vi "write checkpoint report.vi"(8 "error in (no error)":errorcluster, 11 "Autofocus in":refnum<class "Autofocus.lvclass">) -> (0 "error out":errorcluster, 3 "Autofocus out":refnum<class "Autofocus.lvclass">)   [LabVIEW 2012, in "Autofocus.lvclass"]
uses:
  Autofocus.lvclass
  Autofocus.lvclass/Autofocus.ctl
  <vilib>/Utility/file.llb/Write To Spreadsheet File (DBL).vi
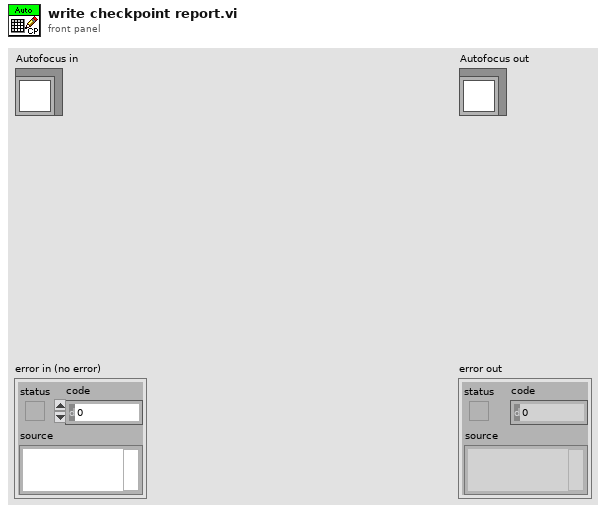
[diagram p1: front panel]
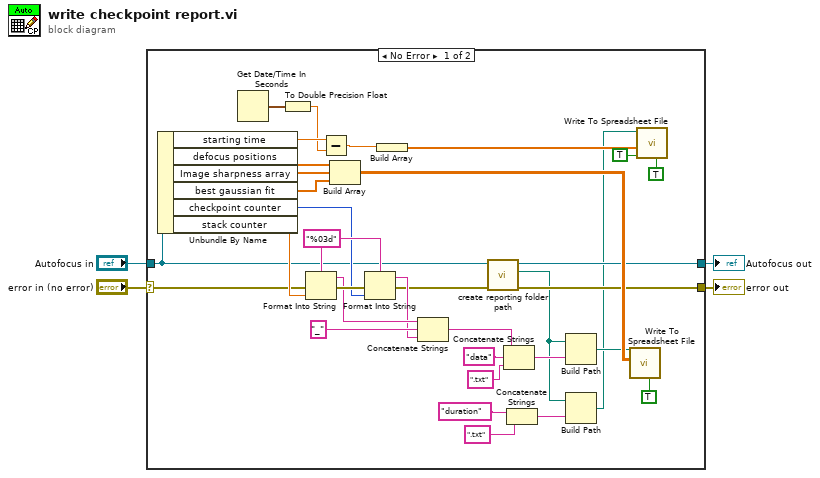
[diagram p0: block diagram]
diagram:
  n1 = case shown="No Error" "error in (no error)" {
    selector: "error in (no error)" -> [w16 w40]
    tunnel: [w11 w40] -> w3
    tunnel: [w12 w39] -> w1
    tunnel: "Autofocus in" -> [w13 w39]
    frame No Error {
      w36 = "%03d" ("format string")
      n2 = Unbundle By Name(w13) -> ("starting time"=w6:dbl, "defocus positions"=w30:dbl[], "Image sharpness array"=w29:dbl[], "best gaussian fit"=w28:dbl[], "checkpoint counter"=w35:i32, "stack counter"=w37:dbl)
      n3 = Get Date/Time In Seconds() -> (seconds since 1Jan1904=w8:timestamp)
      n4 = To Double Precision Float(number=w8) -> (double precision float=w5:dbl)
      n5 = Format Into String(format string=w36, error in=w16, w37) -> (resulting string=w33:string, error out=w38:errorcluster)  [unwired: 1 in]
      n6 = Subtract(x=w6, y=w5) -> (x-y=w7:dbl)
      n7 = Build Array(w30, w29, w28) -> (w27:dbl[][])
      n8 = Format Into String(format string=w36, error in=w38, w35) -> (resulting string=w32:string, error out=w14:errorcluster)  [unwired: 1 in]
      n9 = Build Array(w7) -> (w25:dbl[])
      n10 = Concatenate Strings(w33, "_" ("string"), w32) -> (w15:string)
      n11 = call-dynamic "create reporting folder path.vi"("error in (no error)"=w14, "Autofocus in"=w13) -> ("error out"=w11:errorcluster, "folder base"=w10:path, "Autofocus out"=w12:refnum<class "Autofocus.lvclass">)  [unwired: 6 in, 1 out]
      n12 = Concatenate Strings(w15, "data" ("string"), ".txt" ("string")) -> (w22:string)
      n13 = Concatenate Strings("duration" ("string"), ".txt" ("string")) -> (w17:string)
      n14 = Build Path(base path=w10, name or relative path=w22) -> (appended path=w23:path)
      n15 = Build Path(base path=w10, name or relative path=w17) -> (appended path=w9:path)
      n16 = call-poly <vilib>:"Write To Spreadsheet File.vi"("transpose? (no:F)"=TRUE, "2D data"=w27, "file path (dialog if empty)"=w23) -> ()  [unwired: 5 in, 1 out]
      n17 = call-poly <vilib>:"Write To Spreadsheet File.vi"("transpose? (no:F)"=TRUE, "append to file? (new file:F)"=TRUE, "1D data"=w25, "file path (dialog if empty)"=w9) -> ()  [unwired: 4 in, 1 out]
    }
    frame Error {
    }
  }
  "error out" <- w3
  "Autofocus out" <- w1
